vi "FPGA myRIO Ultrasound (Left).vi"(8 "stop":bool) -> (2 "Object Range (cm)":dbl)   [LabVIEW 2017]
uses:
  <vilib>/myRIO/Instrument Drivers/Onboard IO/DIO/typedefs/DIO Reference.ctl
  <vilib>/myRIO/Common/Instrument Driver Framework/Utilities/typedefs/myRIO Generic Hardware Reference.ctl
  <vilib>/myRIO/Common/Instrument Driver Framework/Utilities/typedefs/Hardware Version Enum.ctl
  <vilib>/myRIO/Common/Instrument Driver Framework/Utilities/typedefs/myRIO v1.0 Reference.ctl
  <vilib>/myRIO/Common/Instrument Driver Framework/Utilities/typedefs/Generic FPGA Reference.ctl
  <vilib>/myRIO/Common/Instrument Driver Framework/myRIO v1.0/DIO/typedefs/DIO Channels List.ctl
  <vilib>/myRIO/Common/Instrument Driver Framework/myRIO v1.0/DIO/typedefs/DIO Channels Enum.ctl
  <vilib>/userdefined/High Color/nirio_resource_hc.ctl
  <vilib>/myRIO/Instrument Drivers/Onboard IO/DIO/vis/Write.vi
  <vilib>/myRIO/Common/Instrument Driver Framework/myRIO v1.0/DIO/vis/myRIO v1.1 Open DIO.vi
  <vilib>/myRIO/Common/Instrument Driver Framework/Utilities/vis/Is FPGA Ref Available.vi
  <vilib>/myRIO/Instrument Drivers/Onboard IO/DIO/vis/Read.vi
  <vilib>/myRIO/Common/Instrument Driver Framework/Utilities/vis/Validate Channels.vi
  <vilib>/myRIO/Common/Instrument Driver Framework/myRIO v1.0/DIO/vis/myRIO v1.0 Reserve DIO.vi
  <vilib>/myRIO/Common/Instrument Driver Framework/myRIO v1.0/Resource Manager/vis/myRIO v1.0 Reserve Channel List.vi
  <vilib>/myRIO/Common/Instrument Driver Framework/myRIO v1.0/DIO/vis/myRIO v1.0 Build MUX Configuration DIO.vi
  <vilib>/myRIO/Common/Instrument Driver Framework/myRIO v1.0/Resource Manager/vis/myRIO v1.0 Reserve Channel.vi
  <vilib>/myRIO/Common/Instrument Driver Framework/myRIO v1.0/Resource Manager/vis/myRIO v1.0 Unreserve Channel.vi
  <vilib>/myRIO/Common/Instrument Driver Framework/myRIO v1.0/Resource Manager/vis/myRIO v1.0 Create Configuration List.vi
  <vilib>/myRIO/Common/Instrument Driver Framework/myRIO v1.0/Resource Manager/vis/myRIO v1.0 Build Mutex Name.vi
  <vilib>/myRIO/Common/Instrument Driver Framework/myRIO v1.0/DIO/vis/myRIO v1.0 Write DIO.vi
  <vilib>/Utility/error.llb/Error Cluster From Error Code.vi
  <vilib>/myRIO/Common/Instrument Driver Framework/myRIO v1.0/myRIO v1.0 Close.vi
  <vilib>/myRIO/Common/Instrument Driver Framework/myRIO v1.0/Resource Manager/vis/myRIO v1.0 Configure IO.vi
  <vilib>/myRIO/Common/Instrument Driver Framework/Utilities/vis/IO Manager.vi
  <vilib>/myRIO/Common/Instrument Driver Framework/Utilities/vis/Configuration Manager.vi
  <vilib>/myRIO/Common/Instrument Driver Framework/myRIO v1.0/myRIO v1.1 Open.vi
  <vilib>/Utility/VariantDataType/GetNumericInfo.vi
  ultrasonic_global.vi
  <vilib>/myRIO/Common/Instrument Driver Framework/myRIO v1.0/DIO/vis/myRIO v1.0 Read DIO.vi
  <vilib>/Analysis/3filter.llb/Butterworth Filter (DBL).vi
  <vilib>/myRIO/Instrument Drivers/Onboard IO/DIO/vis/myRIO DIO Open.xnode
  <vilib>/myRIO/Express VI/Onboard IO/DO/DO Express VI.xnode
  <vilib>/myRIO/Express VI/Onboard IO/DI/DI Express VI.xnode
  <vilib>/myRIO/Instrument Drivers/Onboard IO/DIO/DIO.lvlib
  <vilib>/Analysis/NI_AALBase.lvlib
panel:
  out "Waveform Chart":dbl(graph)
  in  "Trigger pulse interval (mSec)":u32=200
  out "Time of flight (uS)":u32
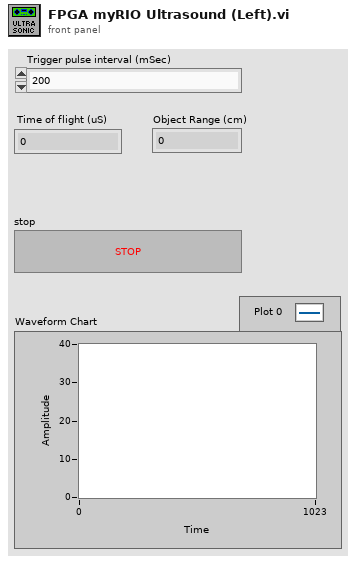
[diagram p1: front panel]
types:
  T1 = typedef "DIO.lvlib/DIO Reference.ctl" = cluster{"myRIO Reference":T2, "DIO Channels List":T6}
  T2 = typedef "myRIO Generic Hardware Reference.ctl" = cluster{"myRIO Model":T3, "myRIO Hardware Reference":T4}
  T3 = typedef "Hardware Version Enum.ctl" = enum16{"Unknown", "myRIO-1900", "myRIO-1950", "roboRIO", "NI ELVIS RIO CM"}
  T4 = typedef "myRIO v1.0 Reference.ctl" = cluster{"Generic FPGA Reference":T5, "Allow multiple opens":bool}
  T5 = typedef "Generic FPGA Reference.ctl" = refnum<k20>
  T6 = typedef "DIO Channels List.ctl" = T7[]
  T7 = typedef "DIO Channels Enum.ctl" = enum16{"Not Connected", "C/DIO0", "C/DIO1", "C/DIO2", "C/DIO3", "C/DIO4", "C/DIO5", "C/DIO6", "C/DIO7", "A/DIO0", "A/DIO1", "A/DIO2", "A/DIO3", "A/DIO4", "A/DIO5", "A/DIO6", "A/DIO7", "A/DIO8", "A/DIO9", "A/DIO10", "A/DIO11", "A/DIO12", "A/DIO13", "A/DIO14", "A/DIO15", "B/DIO0", "B/DIO1", "B/DIO2", "B/DIO3", "B/DIO4", "B/DIO5", "B/DIO6", "B/DIO7", "B/DIO8", "B/DIO9", "B/DIO10", "B/DIO11", "B/DIO12", "B/DIO13", "B/DIO14", "B/DIO15", "LED0", "LED1", "LED2", "LED3", "Button0", "DIO/DIO0", "DIO/DIO1", "DIO/DIO2", "DIO/DIO3", "DIO/DIO4", "DIO/DIO5", "DIO/DIO6", "DIO/DIO7", "DIO/DIO8", "DIO/DIO9", "SPI/CS0", "SPI/CS1", "SPI/CS2", "SPI/CS3", "LED RADIO (Green)", "LED RADIO (Red)", "LED COMM (Green)", "LED COMM (Red)", "LED MODE (Green)", "LED MODE (Red)"}
  T8 = typedef "nirio_resource_hc.ctl" = tag
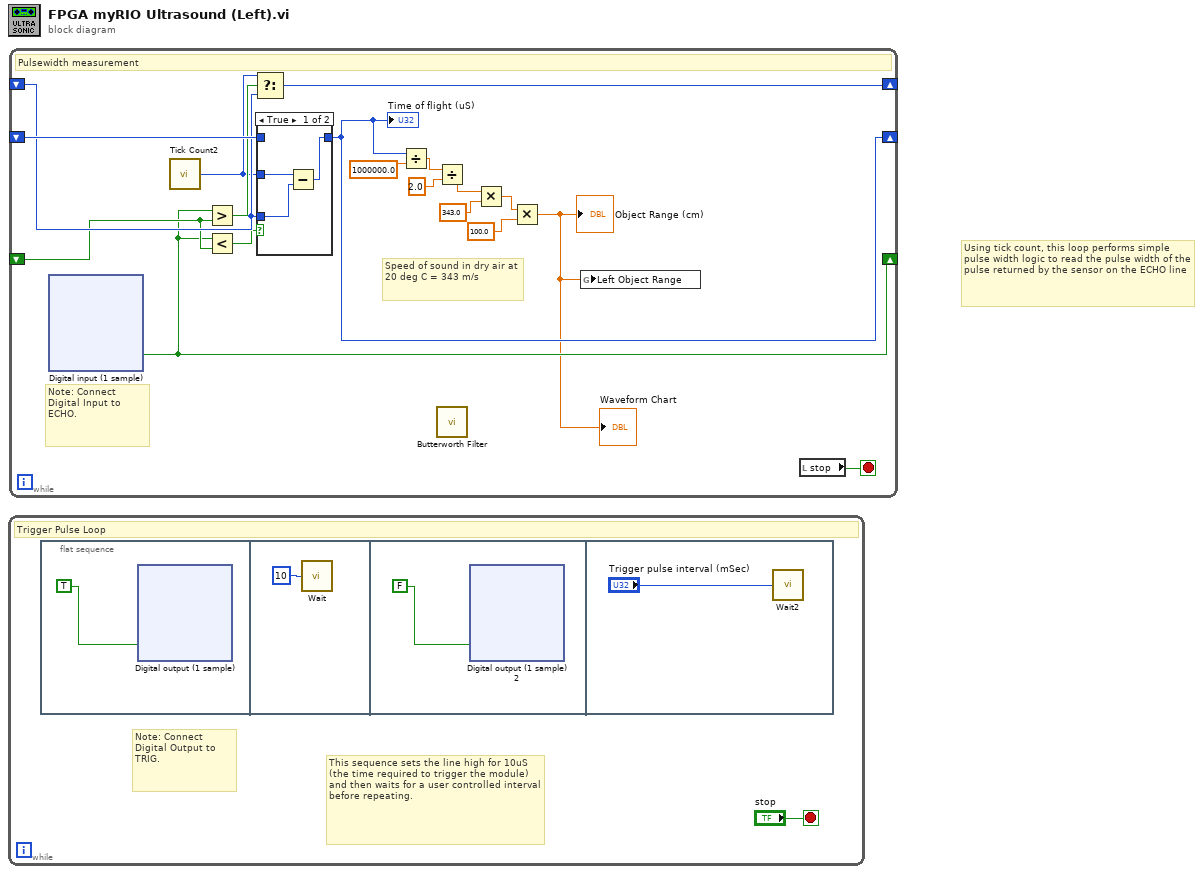
[diagram p0: block diagram]
diagram:
  # "Using tick count, this loop performs simple pulse width logic to read the pulse width of the pulse returned by the sensor on the ECHO line"
  n1 = while {
    stop <- "stop" stop-if-true
    # "Note: Connect Digital Output to TRIG."
    # "This sequence sets the line high for 10uS (the time required to trigger the module) and then waits for a user controlled interval before repeating."
    # "Trigger Pulse Loop"
    n2 = flat-sequence {
      frame #0 {
        n3 = xnode "Digital output (1 sample)"("A/DIO4 (Pin 19)"=TRUE ("ConnectorC/DIO6")) -> ()  [unwired: 1 in, 1 out]
      }
      frame #1 {
        n4 = call "Wait"("Count(uSec)"=u32 10) -> ()  [unwired: 1 out]
      }
      frame #2 {
        n5 = xnode "Digital output (1 sample) 2"("A/DIO4 (Pin 19)"=FALSE ("ConnectorC/DIO6")) -> ()  [unwired: 1 in, 1 out]
      }
      frame #3 {
        n6 = call "Wait2"("Count(mSec)"="Trigger pulse interval (mSec)") -> ()  [unwired: 1 out]
      }
    }
  }
  n7 = while "Pulsewidth Measurement + Sound Output" {
    shift-left: _ -> [w93]
    shift-right: [w84] -> _
    shift-left: _ -> [w92]
    shift-right: [w91] -> _
    shift-left: _ -> [w89]
    shift-right: [w77] -> _
    stop <- w86 stop-if-true
    # "Note: Connect Digital Input to ECHO."
    # "Speed of sound in dry air at 20 deg C = 343 m/s"
    # "Pulsewidth measurement"
    n8 = xnode "Digital input (1 sample)"() -> ("A/DIO5 (Pin 21)"=w77:bool)  [unwired: 1 in, 1 out]
    n9 = call "Tick Count2"() -> ("Tick Count(uSec)"=w87:u32)
    n10 = Greater?(x=w77, y=w89) -> (0:w90:bool)
    n11 = Less?(x=w77, y=w89) -> (x < y?=w88:bool)
    n12 = Select(t=w87, s=w90, f=w92) -> (s? t:f=w91:u32)
    n13 = case shown="True" w88 {
      tunnel: w93 -> [_ w132]
      tunnel: w87 -> [w129 _]
      tunnel: w92 -> [w130 _]
      tunnel: [w131 w132] -> w84
      frame True {
        n14 = Subtract(x=w129, y=w130) -> (x-y=w131:u32)
      }
      frame False {
      }
    }
    "Time of flight (uS)" <- w84
    n15 = Divide(x=w84, y=1000000.0) -> (x/y=w83:dbl)
    n16 = Divide(x=w83, y=2.0) -> (x/y=w81:dbl)
    n17 = call-poly <vilib>:"Butterworth Filter.vi"() -> ()  [unwired: 8 in, 2 out]
    n18 = Multiply(x=w81, y=343.0) -> (x*y=w79:dbl)
    n19 = Multiply(x=w79, y=100.0) -> (x*y=w76:dbl)
    "Object Range (cm)" <- w76
    "Waveform Chart" <- w76
    n20 = global write "ultrasonic_global.vi" "Left Object Range"(w76) -> ()
    n21 = local read "stop"() -> (w86:bool)
  }
